vi "模块启用配置框.vi"() -> ()   [LabVIEW 2016]
uses:
  <vilib>/Utility/config.llb/NI_LVConfig.lvlib
panel:
  out "配置文件 path":path
  out "ping":bool
  in  "超标留样启用":bool caption="质控单元禁用"
  in  "总氮启用":bool caption="总磷总氮禁用"
  in  "取消":bool
  in  "确认":bool
  in  "CODMn启用":bool caption="CODMn禁用"
  in  "质控单元启用":bool caption="质控单元禁用"
  in  "总磷启用":bool caption="总磷总氮禁用"
  in  "流量计启用":bool caption="流量计禁用"
  in  "氨氮启用":bool caption="氨氮禁用"
  in  "多参数启用":bool caption="多参数禁用"
  in  "CODcr启用":bool caption="CODcr禁用"
  # "模块启用配置"
  # "说明:\n选择所需要启动的模块,并按确认,软件将重启生效."
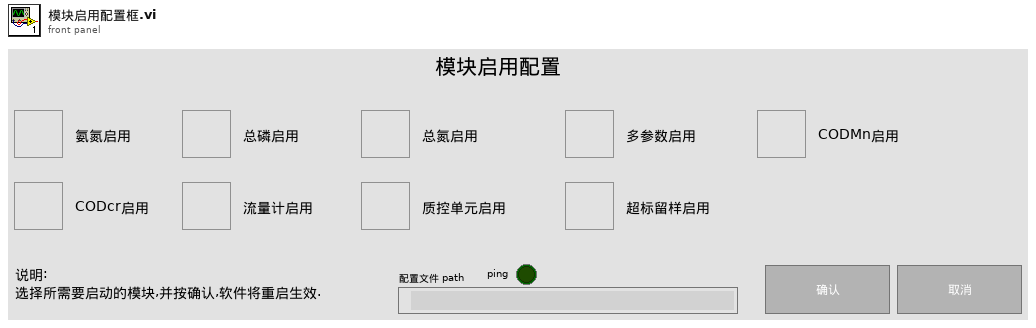
[diagram p1: front panel]
types:
  T1 = typedef "NI_LVConfig.lvlib/Config Data RefNum.ctl" = refnum<k1>
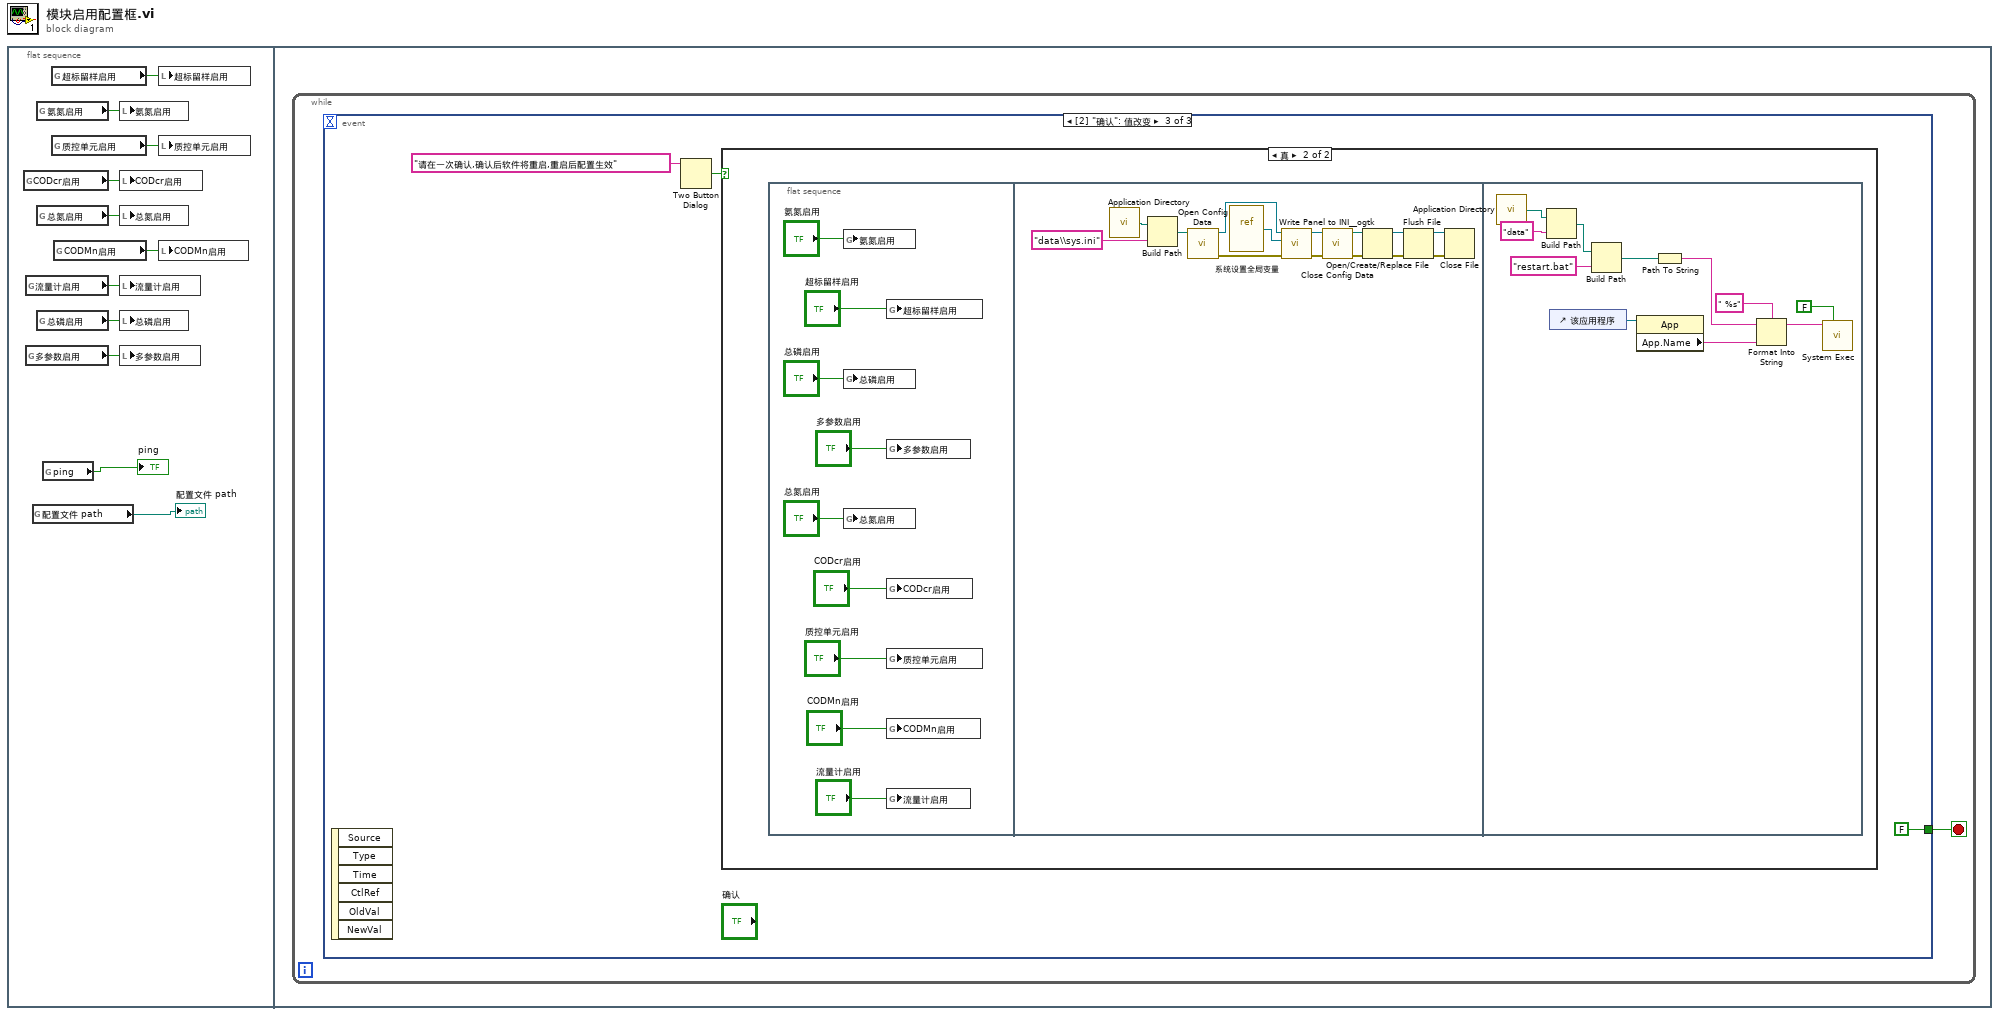
[diagram p0: block diagram]
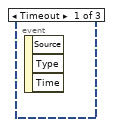
[diagram p2: hidden frame]
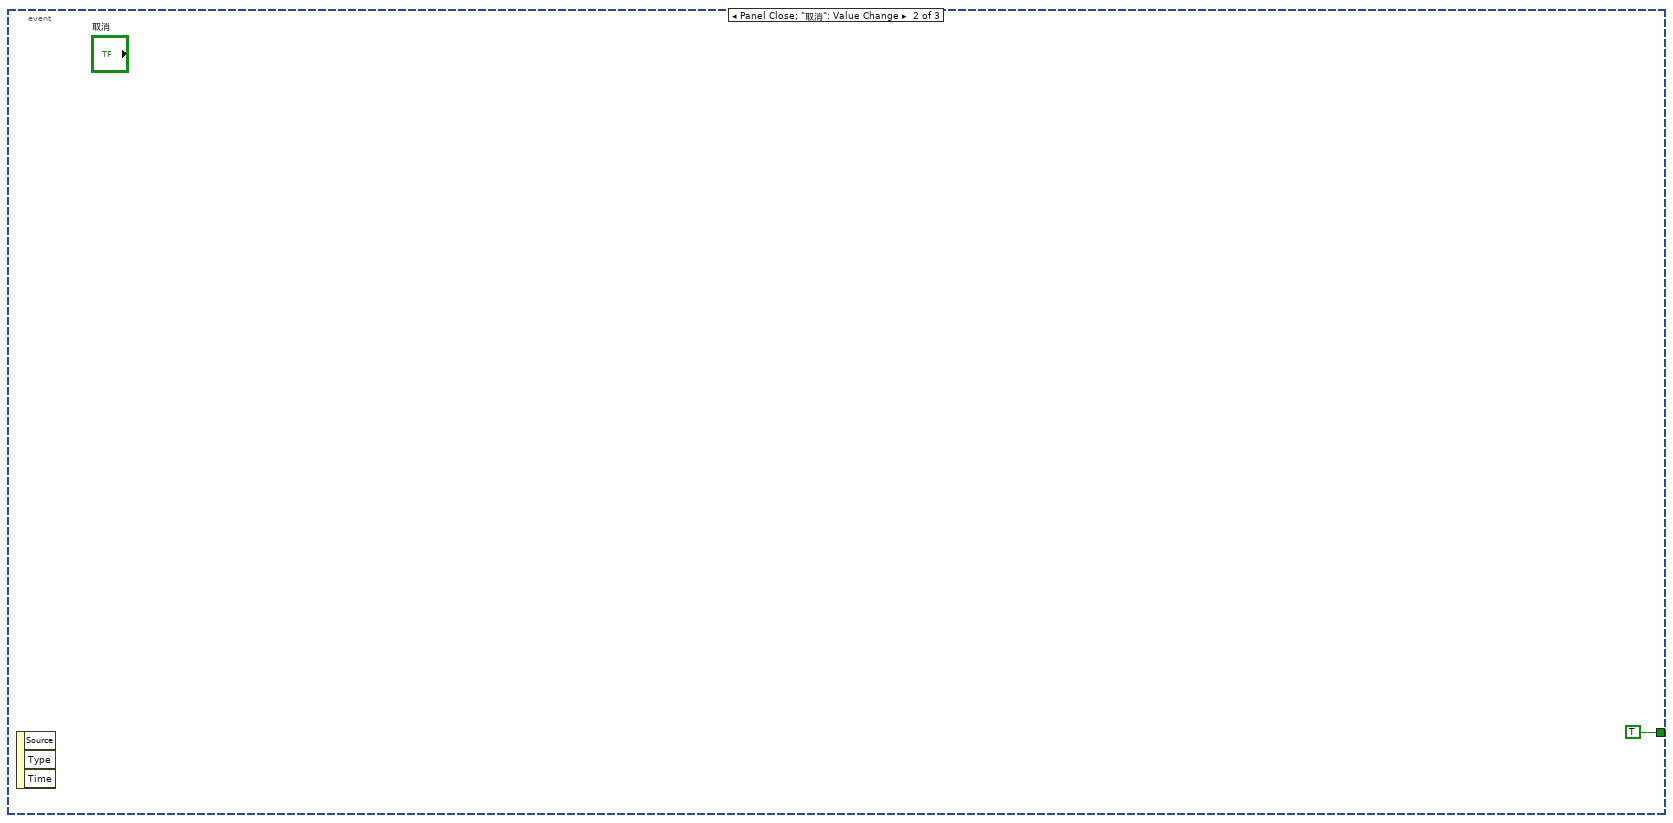
[diagram p3: hidden frame]
diagram:
  n1 = flat-sequence {
    frame #0 {
      n2 = global read "系统设置全局变量.vi" "CODcr启用"() -> (w11:bool)
      n3 = global read "系统设置全局变量.vi" "流量计启用"() -> (w8:bool)
      n4 = global read "系统设置全局变量.vi" "多参数启用"() -> (w9:bool)
      n5 = global read "ping全局.vi" "配置文件 path"() -> (→"配置文件 path":path)
      n6 = global read "系统设置全局变量.vi" "氨氮启用"() -> (w7:bool)
      n7 = global read "系统设置全局变量.vi" "总氮启用"() -> (w4:bool)
      n8 = global read "系统设置全局变量.vi" "总磷启用"() -> (w10:bool)
      n9 = global read "ping全局.vi" "ping"() -> (→"ping":bool)
      n10 = global read "系统设置全局变量.vi" "超标留样启用"() -> (w3:bool)
      n11 = global read "系统设置全局变量.vi" "质控单元启用"() -> (w5:bool)
      n12 = global read "系统设置全局变量.vi" "CODMn启用"() -> (w6:bool)
      n13 = local write "氨氮启用"(w7) -> ()
      n14 = local write "CODcr启用"(w11) -> ()
      n15 = local write "总氮启用"(w4) -> ()
      n16 = local write "流量计启用"(w8) -> ()
      n17 = local write "总磷启用"(w10) -> ()
      n18 = local write "多参数启用"(w9) -> ()
      n19 = local write "超标留样启用"(w3) -> ()
      n20 = local write "质控单元启用"(w5) -> ()
      n21 = local write "CODMn启用"(w6) -> ()
    }
    frame #1 {
      n22 = while {
        stop <- w12 stop-if-true
        n23 = event shown="[2] \"确认\": 值改变" {
          selector: _ -> [_ _ _]
          dyn-events: _ -> [_ _ _]
          timeout: _ -> [_ _ _]
          tunnel: [_ TRUE FALSE] -> w12
          event Timeout {
            n24 = event-data() -> ()  [unwired: 1 in, 3 out]
          }
          event Panel Close; "取消": Value Change {
            n25 = event-data() -> ()  [unwired: 1 in, 3 out]
          }
          event "确认": Value Change {
            n26 = event-data() -> ()  [unwired: 1 in, 6 out]
            n27 = Two Button Dialog(message="请在一次确认,确认后软件将重启,重启后配置生效" ("消息")) -> (T button?=w14:bool)  [unwired: 2 in]
            n28 = case shown="真" w14 {
              frame False {
              }
              frame True {
                n29 = flat-sequence {
                  frame #0 {
                    n30 = global write "系统设置全局变量.vi" "氨氮启用"("氨氮启用") -> ()
                    n31 = global write "系统设置全局变量.vi" "总磷启用"("总磷启用") -> ()
                    n32 = global write "系统设置全局变量.vi" "总氮启用"("总氮启用") -> ()
                    n33 = global write "系统设置全局变量.vi" "超标留样启用"("超标留样启用") -> ()
                    n34 = global write "系统设置全局变量.vi" "多参数启用"("多参数启用") -> ()
                    n35 = global write "系统设置全局变量.vi" "CODcr启用"("CODcr启用") -> ()
                    n36 = global write "系统设置全局变量.vi" "质控单元启用"("质控单元启用") -> ()
                    n37 = global write "系统设置全局变量.vi" "CODMn启用"("CODMn启用") -> ()
                    n38 = global write "系统设置全局变量.vi" "流量计启用"("流量计启用") -> ()
                  }
                  frame #1 {
                    n39 = call <vilib>:"Application Directory.vi"() -> ("Application Directory"=w27:path)
                    n40 = Build Path(base path=w27, name or relative path="data\\sys.ini" ("名称或相对路径")) -> (appended path=w26:path)
                    n41 = call <vilib>:"Open Config Data.vi"("configuration file path"=w26) -> ("error out"=w36:errorcluster, "refnum"=w39:T1)  [unwired: 8 in, 1 out]
                    n42 = vi-ref "系统设置全局变量.vi"() -> (w38:refnum<vi>)
                    n43 = call <userlib>:"Write Panel to INI__ogtk.vi"("error in (no error)"=w36, "VI ref"=w38, "refnum"=w39) -> ("error out"=w35:errorcluster, "refnum out"=w37:T1)  [unwired: 7 in]
                    n44 = call <vilib>:"Close Config Data.vi"("error in (no error)"=w35, "refnum"=w37) -> ("error out"=w30:errorcluster, "file path"=w29:path)  [unwired: 8 in]
                    n45 = Open/Create/Replace File(file path (use dialog)=w29, error in=w30) -> (refnum out=w33:refnum<file>, error out=w34:errorcluster)  [unwired: 4 in, 1 out]
                    n46 = Flush File(refnum=w33, error in=w34) -> (refnum out=w32:refnum<file>, error out=w31:errorcluster)
                    n47 = Close File(refnum=w32, error in=w31) -> ()  [unwired: 2 out]
                  }
                  frame #2 {
                    n48 = call <vilib>:"Application Directory.vi"() -> ("Application Directory"=w49:path)
                    n49 = Build Path(base path=w49, name or relative path="data" ("名称或相对路径")) -> (appended path=w47:path)
                    n50 = control-ref of="该应用程序"() -> (w50:refnum<vi>)
                    n51 = Build Path(base path=w47, name or relative path="restart.bat" ("名称或相对路径")) -> (appended path=w45:path)
                    n52 = property class="App"(reference=w50) -> ("App.Name"=w42:string)  [unwired: 1 in, 2 out]
                    n53 = Path To String(path=w45) -> (string=w44:string)
                    n54 = Format Into String(format string=" %s" ("格式字符串"), initial string=w44, w42) -> (resulting string=w41:string)  [unwired: 1 in, 1 out]
                    n55 = call <vilib>:"System Exec.vi"("wait until completion? (T)"=FALSE, "command line"=w41) -> ()  [unwired: 6 in, 4 out]
                  }
                }
              }
            }
          }
        }
      }
    }
  }
